vi "Read next TLV Header.vi"(8 "error in (no error)":errorcluster, 11 "object in":refnum<class "CAN IO.lvclass">) -> (0 "error out":errorcluster, 1 "Length":u8, 2 "Type":u8, 3 "object out":refnum<class "CAN IO.lvclass">)   [LabVIEW 2013, in "CAN IO.lvclass"]
uses:
  CAN IO.lvclass
  CAN IO.lvclass/CAN IO.ctl
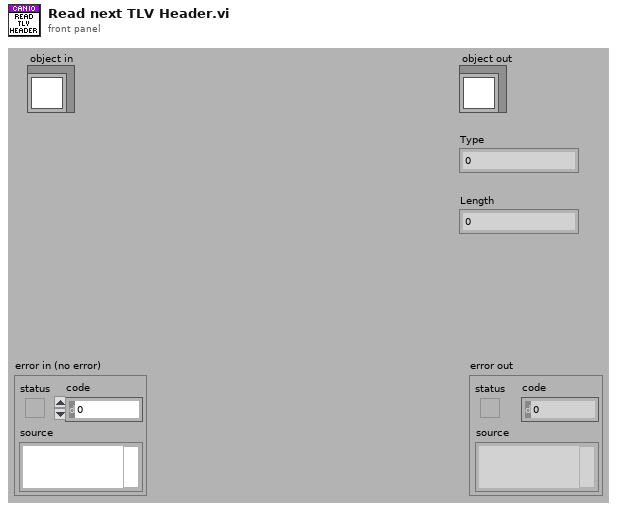
[diagram p1: front panel]
types:
  T1 = enum16{"big-endian, network order", "native, host order", "little-endian"}
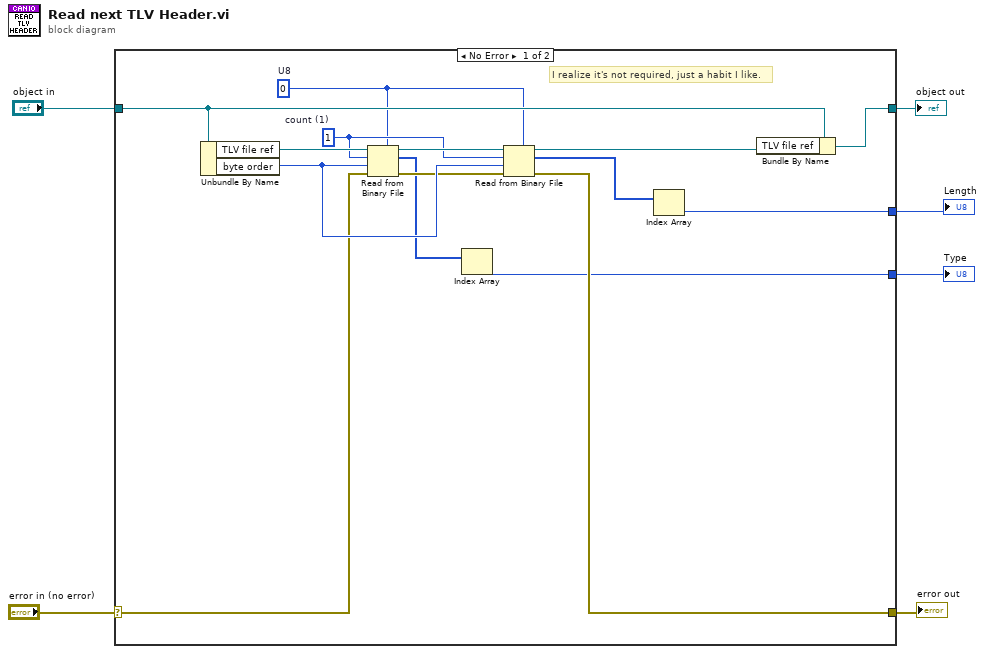
[diagram p0: block diagram]
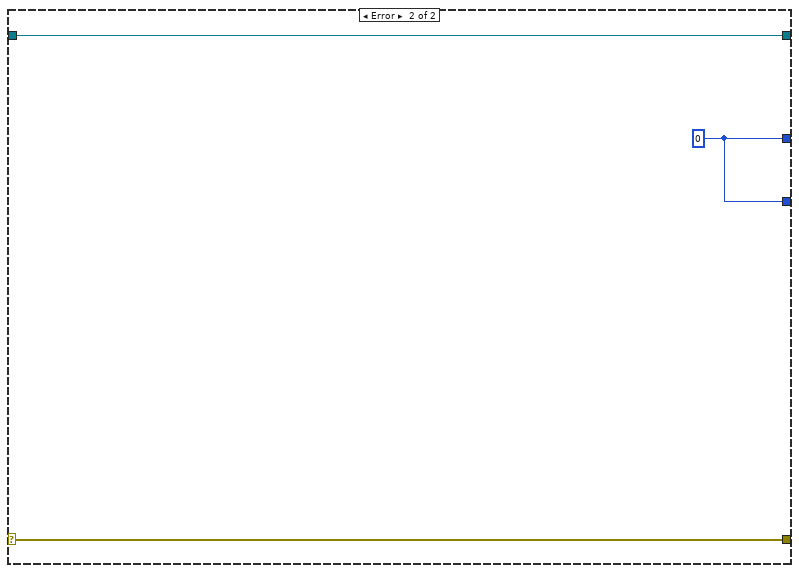
[diagram p2: hidden frame]
diagram:
  n1 = case shown="No Error" "error in (no error)" {
    selector: "error in (no error)" -> [w15 w24]
    tunnel: [w11 w24] -> w5
    tunnel: [w12 w23] -> w3
    tunnel: "object in" -> [w20 w23]
    tunnel: [w9 w22] -> w2
    tunnel: [w7 w22] -> w1
    frame No Error {
      w17 = u8 0  # U8
      w18 = 1  # count (1)
      # "I realize it's not required, just a habit I like."
      n2 = Unbundle By Name(w20) -> ("TLV file ref"=w21:refnum<file>, "byte order"=w16:T1)
      n3 = Read from Binary File(5:w17, 8:w15, 9:w16, 10:w18, 11:w21) -> (0:w14:errorcluster, 2:w10:u8[], 3:w19:refnum<file>)  [unwired: 1 in, 1 out]
      n4 = Index Array(array=w10) -> (element=w9:u8)  [unwired: 1 in]
      n5 = Read from Binary File(5:w17, 8:w14, 9:w16, 10:w18, 11:w19) -> (0:w11:errorcluster, 2:w8:u8[], 3:w13:refnum<file>)  [unwired: 1 in, 1 out]
      n6 = Index Array(array=w8) -> (element=w7:u8)  [unwired: 1 in]
      n7 = Bundle By Name(cluster=w20, "TLV file ref"=w13) -> (w12:refnum<class "CAN IO.lvclass">)
    }
    frame Error {
      w22 = u8 0 ("I32")
    }
  }
  "error out" <- w5
  "object out" <- w3
  "Type" <- w2
  "Length" <- w1
